vi "Write String.vi"(7 "section":string, 8 "error in":errorcluster, 9 "value":string, 10 "key":string, 11 "config file in":refnum<data-value>) -> (0 "error out":errorcluster, 2 "found?":bool, 3 "config file out":refnum<data-value>)   [LabVIEW 2012, in "configlib.lvlib"]
uses:
  configlib.lvlib
  Configuration File Definition.ctl
  File Options.ctl
  Set Key.vi
  Replace Value on Key Line.vi
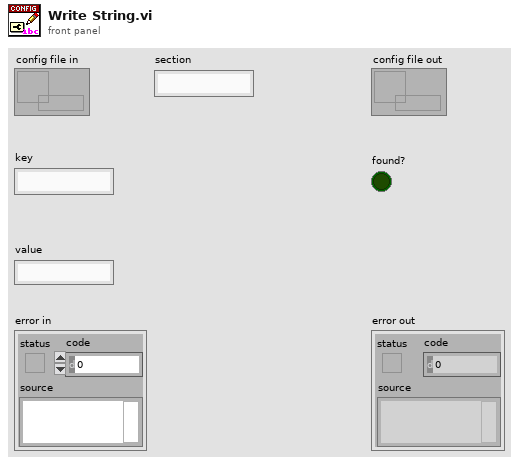
[diagram p1: front panel]
types:
  T1 = typedef "configlib.lvlib/Configuration File Definition.ctl" = cluster{"dirty":bool, "path":path, "Fileopts":T2, "Section Lookup":variant, "Key Lookup":variant, "Raw File":string[]}
  T2 = typedef "configlib.lvlib/File Options.ctl" = cluster{"Name/Value delimiter (\"=\")":string, "Comment delimiter (\";\")":string}
  T3 = typedef "configlib.lvlib/Key Definition.ctl" = cluster{"Line Number":i32, "Value":string}
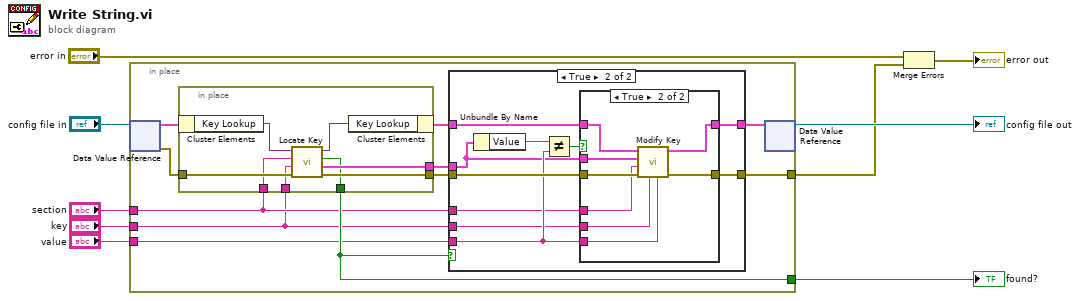
[diagram p0: block diagram]
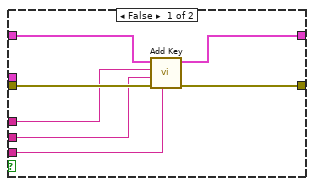
[diagram p2: hidden frame]
diagram:
  n1 = in-place {
    in-place-border: "key" -> [w10]
    in-place-border: "section" -> [w11]
    in-place-border: [w13] -> w4
    in-place-border: [w18] -> w6
    in-place-border: "value" -> [w12]
    n2 = in-place-dvr #1("config file in") -> (w20:T1, w19:errorcluster)
    n3 = in-place {
      in-place-border: w19 -> [w53]
      in-place-border: [w52] -> w16
      in-place-border: [w51] -> w17
      in-place-border: [w50] -> w18
      in-place-border: w10 -> [w49]
      in-place-border: w11 -> [w48]
      n4 = in-place-cluster #2(w20) -> ("Key Lookup"=w55:variant)
      n5 = call "Locate Key.vi"("error in"=w53, "key"=w49, "section"=w48, "key lookup"=w55) -> ("error out"=w52:errorcluster, "key definition"=w51:T3, "found?"=w50:bool, "key lookup out"=w54:variant)  [unwired: 4 in]
      n6 = in-place-cluster #2("Key Lookup"=w54) -> (w15:T1)
    }
    n7 = case shown="True" w18 {
      tunnel: w17 -> [_ w28]
      tunnel: w16 -> [w26 w33]
      tunnel: w15 -> [w22 w35]
      tunnel: [w27 w34] -> w14
      tunnel: [w25 w32] -> w13
      tunnel: w12 -> [w21 w31]
      tunnel: w11 -> [w24 w29]
      tunnel: w10 -> [w23 w30]
      frame False {
        n8 = call "Add Key.vi"("value"=w21, "error in"=w26, "key"=w23, "section"=w24, "Configuration File in"=w22) -> ("error out"=w25:errorcluster, "Configuration File out"=w27:T1)  [unwired: 5 in]
      }
      frame True {
        n9 = Unbundle By Name(w28) -> ("Value"=w37:string)
        n10 = Not Equal?(x=w37, y=w31) -> (x != y?=w36:bool)
        n11 = case shown="True" w36 {
          tunnel: w35 -> [w39 w46]
          tunnel: [w39 w47] -> w34
          tunnel: w33 -> [w38 w45]
          tunnel: [w38 w44] -> w32
          tunnel: w31 -> [_ w43]
          tunnel: w30 -> [_ w42]
          tunnel: w29 -> [_ w41]
          tunnel: w28 -> [_ w40]
          frame False {
            # "no change"
          }
          frame True {
            n12 = call "Modify Key.vi"("value"=w43, "key"=w42, "error in"=w45, "section"=w41, "key definition"=w40, "Configuration File in"=w46) -> ("error out"=w44:errorcluster, "Configuration File out"=w47:T1)  [unwired: 4 in]
          }
        }
      }
    }
    n13 = in-place-dvr #1(w14) -> (→"config file out":refnum<data-value>)  [unwired: 1 out]
  }
  "found?" <- w6
  n14 = Merge Errors("error in", w4) -> (→"error out":errorcluster)
